vi "timer.vi"(8 "error in":errorcluster, 10 "timerstate":T1, 11 "limit":dbl) -> (0 "error out":errorcluster, 2 "elapsed":dbl, 3 "limit out":bool)   [LabVIEW 2015]
uses:
  controls/timerstate.ctl
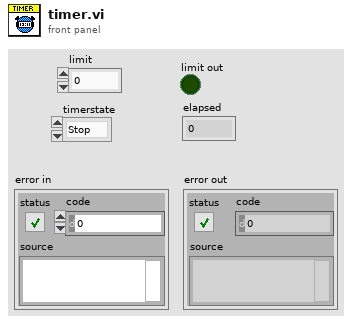
[diagram p1: front panel]
types:
  T1 = typedef "timerstate.ctl" = enum16{"Stop", "Start"}
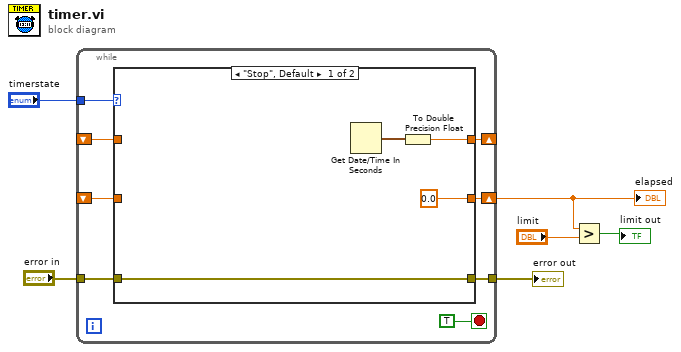
[diagram p0: block diagram]
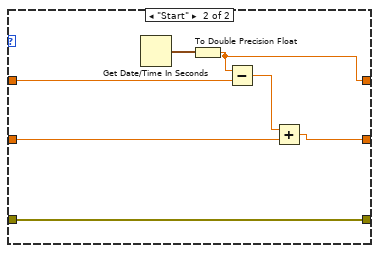
[diagram p2: hidden frame]
diagram:
  n1 = while {
    tunnel: "timerstate" -> [w13]
    shift-right: [w12] -> _
    shift-left: _ -> [w10]
    shift-right: [w11] -> w5
    shift-left: _ -> [w9]
    tunnel: "error in" -> [w8]
    tunnel: [w7] -> w1
    stop <- TRUE stop-if-true
    n2 = case shown="\"Stop\", Default" w13 {
      tunnel: [w17 w20] -> w12
      tunnel: [0.0 w21] -> w11
      tunnel: w10 -> [_ w24]
      tunnel: w9 -> [_ w22]
      tunnel: w8 -> [w15 w19]
      tunnel: [w15 w19] -> w7
      frame "Stop", Default {
        n3 = Get Date/Time In Seconds() -> (seconds since 1Jan1904=w18:timestamp)
        n4 = To Double Precision Float(number=w18) -> (double precision float=w17:dbl)
      }
      frame "Start" {
        n5 = Get Date/Time In Seconds() -> (seconds since 1Jan1904=w25:timestamp)
        n6 = To Double Precision Float(number=w25) -> (double precision float=w20:dbl)
        n7 = Subtract(x=w20, y=w24) -> (x-y=w23:dbl)
        n8 = Add(x=w23, y=w22) -> (x+y=w21:dbl)
      }
    }
  }
  "elapsed" <- w5
  "error out" <- w1
  n9 = Greater?(x=w5, y="limit") -> (0:→"limit out":bool)
